vi "read_from_socket_01.vi"(4 "error out":errorcluster, 5 "Reader ID":string, 6 "correct answer":string, 7 "In connection ID":refnum<k5>) -> (0 "warning out":errorcluster, 2 "answer":string, 3 "Out connection ID":refnum<k5>)   [LabVIEW 2010]
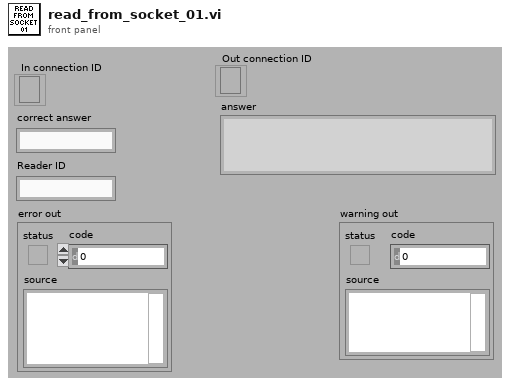
[diagram p1: front panel]
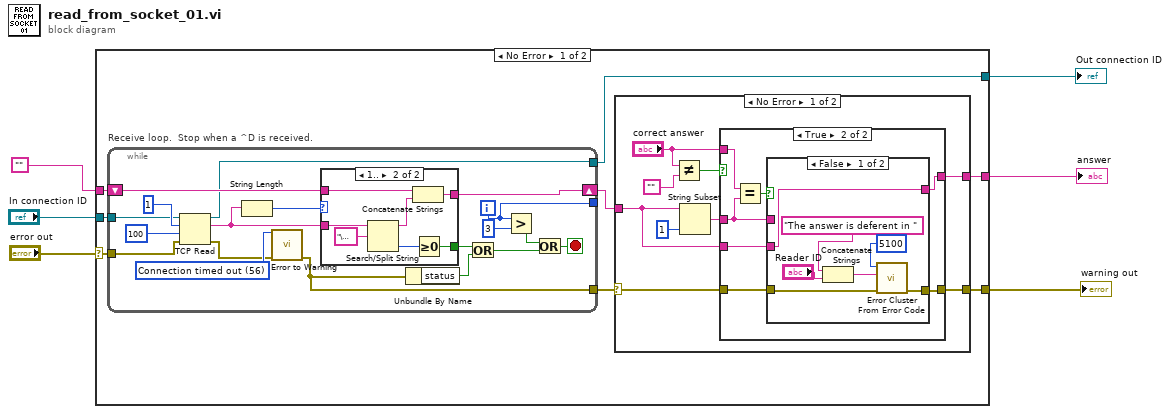
[diagram p0: block diagram]
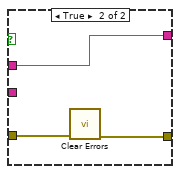
[diagram p3: hidden frame]
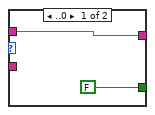
[diagram p5: hidden frame]
diagram:
  n1 = case shown="No Error" "error out" {
    selector: "error out" -> [w7 w73]
    tunnel: "In connection ID" -> [w14 w74]
    tunnel: [w13 w74] -> w5
    tunnel: [w11 w75] -> w4
    tunnel: [w10 w73] -> w3
    tunnel: "" -> [w8 w75]
    frame No Error {
      n2 = while "Receive loop.  Stop when a ^D is received." {
        shift-left: w8 -> [w60]
        shift-right: [w59] -> w12
        tunnel: [w47] -> w9
        tunnel: w14 -> [w61]
        tunnel: [w49] -> _
        tunnel: w7 -> [w46]
        tunnel: [w45] -> w13
        i -> [w49]
        stop <- w52 stop-if-true
        w55 = 56 items=["No Error", "Argument Error", "Memory Full", "Out of Zone", "End of File", "File Already Open", "Generic File IO Error", "File Not Found", "File Permission Error", "Disk Full", "Duplicate Path", "Too Many Files Open", "Not Enabled", "Resource File Not Found", "Cannot Add Resource", "Resource Not Found", "Image Not Found", "Image Memory Error", "Pen Does Not Exist", "Config Bad Type", "Config Token Not Found", "Config Parse Error", "Config Memory Error", "Bad External Code Format", "Bad External Code Offset", "External Code Not Present", "Null Window", "Destroy Window Mixup", "Null Menu", "Print Aborted", "Bad Print Record", "Print Driver Error", "Windows Error During Print", "Memory Error During Print", "Print Dialog Error", "Generic Print Error", "Invalid Device Refnum", "Device Not Found", "Device Parameter Error", "Device Unit Error", "Can't Open Device", "Device Call Aborted", "Generic Error", "Cancelled By User", "Object ID Too Low", "Object ID Too High", "Object Not In Heap", "Unknown Heap", "Bad DefProc ID", "DefProc Not In Table", "Message Out Of Range", "Null Method", "Unknown Message", "Manager Call Not Supported", "Bad address", "Connection In progress", "Connection timed out", "Connection is already in progress", "Network attribute not supported", "Network error", "Address in use", "System out of memory", "Connection aborted", "Connection refused", "Connection is not connected", "Connection is already connected", "Connection closed", "Initialize error (interapplication manager)", "Bad occurrence", "Wait on unbound occurrence handler", "Occurrence queue overflow", "Bad path", "Semaphore not signaled", "Unrecognized type (interapplication manager)"] ("1st Error to Convert")
        n3 = TCP Read(connection ID=w61, bytes to read=1, error in (no error)=w46, 9:100) -> (connection ID out=w45:refnum<k5>, data out=w58:string, error out=w48:errorcluster)  [unwired: 1 in]
        n4 = String Length(string=w58) -> (length=w63:i32)
        n5 = call <vilib>:"Error to Warning.vi"("1st Error to Convert"=w55, "error in"=w48) -> ("warning out"=w47:errorcluster)  [unwired: 13 in]
        n6 = case shown="1.." w63 {
          tunnel: w58 -> [_ w69]
          tunnel: w60 -> [w65 w72]
          tunnel: [w65 w71] -> w59
          tunnel: [FALSE w66] -> w57
          frame ..0 {
          }
          frame 1.. {
            n7 = Search/Split String(string=w69, search string/char (-)="\u0004") -> (substring before match=w68:string, offset of match=w67:i32)  [unwired: 1 in, 1 out]
            n8 = Concatenate Strings(w72, w68) -> (w71:string)
            n9 = Greater Or Equal To 0?(x=w67) -> (x >= 0?=w66:bool)
          }
        }
        n10 = Unbundle By Name(w47) -> ("status"=w54:bool)
        n11 = Or(x=w57, y=w54) -> (x .or. y?=w53:bool)
        n12 = Greater?(x=w49, y=3) -> (0:w51:bool)
        n13 = Or(x=w51, y=w53) -> (x .or. y?=w52:bool)
      }
      n14 = case shown="No Error" w9 {
        selector: w9 -> [w18 w44]
        tunnel: w12 -> [w15 w43]
        tunnel: [w21 w43] -> w11
        tunnel: [w20 w44] -> w10
        frame No Error {
          n15 = Not Equal?(x="correct answer", y="") -> (x != y?=w22:bool)
          n16 = String Subset(string=w15, length (rest)=1 ("length (rest)")) -> (substring=w16:string)  [unwired: 1 in]
          n17 = case shown="True" w22 {
            tunnel: w16 -> [w25 w26]
            tunnel: [w25 w29] -> w21
            tunnel: [w24 w30] -> w20
            tunnel: w18 -> [w24 w31]
            tunnel: "correct answer" -> [_ w28]
            tunnel: w15 -> [_ w27]
            frame False {
            }
            frame True {
              n18 = Equal?(x=w28, y=w26) -> (x = y?=w32:bool)
              n19 = case shown="False" w32 {
                tunnel: w31 -> [w38 w42]
                tunnel: [w39 w41] -> w30
                tunnel: [w33 w40] -> w29
                tunnel: w27 -> [w33 _]
                tunnel: w26 -> [_ w40]
                frame False {
                  n20 = Concatenate Strings("The answer is deferent in ", "Reader ID") -> (w34:string)
                  n21 = call <vilib>:"Error Cluster From Error Code.vi"("error in (no error)"=w38, "error message (\"\")"=w34, "error code (0)"=5100) -> ("error out"=w39:errorcluster)  [unwired: 6 in]
                }
                frame True {
                  n22 = call <vilib>:"Clear Errors.vi"("error in (no error)"=w42) -> ("error out"=w41:errorcluster)  [unwired: 6 in]
                }
              }
            }
          }
        }
        frame Error {
        }
      }
    }
    frame Error {
    }
  }
  "answer" <- w4
  "warning out" <- w3
  "Out connection ID" <- w5
